vi "Run.vi"(8 "error in (no error)":errorcluster, 11 "Pub Sub Message Channel in":refnum<class "Pub Sub Message Channel.lvclass">) -> (0 "error out":errorcluster, 3 "Pub Sub Message Channel out":refnum<class "Pub Sub Message Channel.lvclass">)   [LabVIEW 2020, in "Actor Pub Sub Channels.lvlib" / "Pub Sub Message Channel.lvclass"]
uses:
  Pub Sub Message Channel.lvclass
  Close Channel Message/Close Channel Message.lvclass
  Pub Sub Message Channel.lvclass/Pub Sub Message Channel.ctl
  <vilib>/ActorFramework/Message Queue/Message Queue.lvclass/Message Queue.ctl
  <vilib>/ActorFramework/Message Dequeuer/Message Dequeuer.lvclass/Message Dequeuer.ctl
  <vilib>/ActorFramework/Message Priority Queue/Priority Dequeue.vi
  <vilib>/ActorFramework/Message Queue/Message Queue.lvclass
  <vilib>/ActorFramework/Message Dequeuer/Message Dequeuer.lvclass
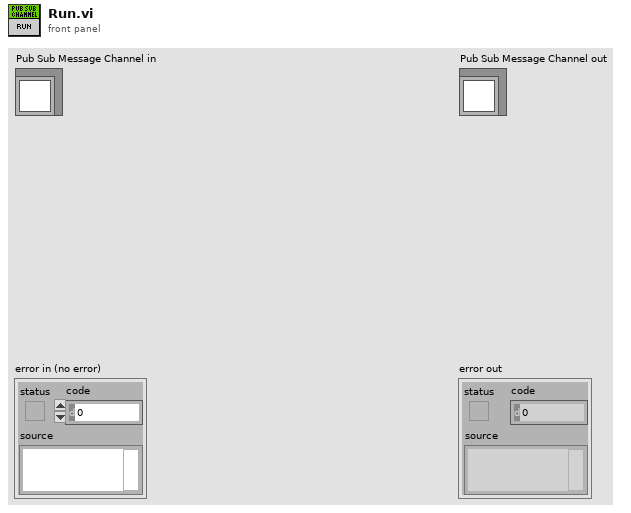
[diagram p1: front panel]
types:
  T1 = typedef "Actor Framework.lvlib/Message Dequeuer.lvclass/Dequeue Priority.ctl" = enum16{"Low", "Normal", "High", "Critical"}
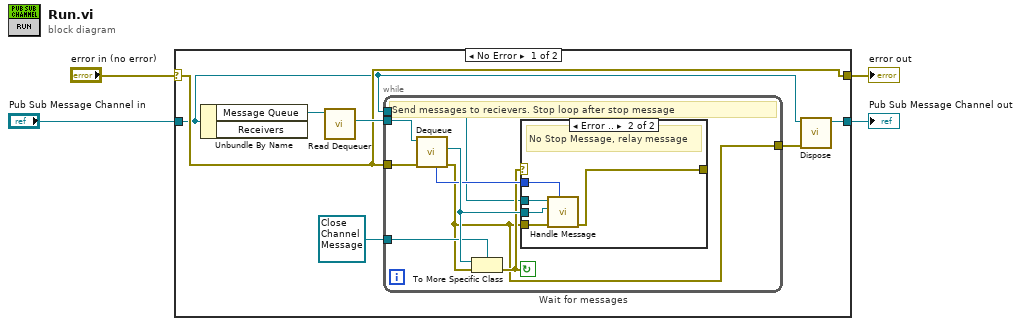
[diagram p0: block diagram]
diagram:
  n1 = case shown="No Error" "error in (no error)" {
    selector: "error in (no error)" -> [w10 w27]
    tunnel: [w10 w27] -> w3
    tunnel: [w5 w26] -> w1
    tunnel: "Pub Sub Message Channel in" -> [w6 w26]
    frame No Error {
      n2 = Unbundle By Name(w6) -> ("Message Queue"=w8:refnum<class "Message Queue.lvclass">)  [unwired: 1 out]
      n3 = call <vilib>:"Read Dequeuer.vi"("Message Queue"=w8) -> ("Message Dequeuer"=w11:refnum<class "Message Dequeuer.lvclass">)  [unwired: 10 in]
      n4 = while "Wait for messages" {
        tunnel: w11 -> [w19]
        tunnel: w10 -> [w18]
        tunnel: [w12] -> w9
        tunnel: refnum<class "Close Channel Message.lvclass"> refnum ("Actor Pub Sub Channels.lvlib:Close Channel Message.lvclass") -> [w15]
        tunnel: w6 -> [w13]
        stop <- w14 continue-if-true
        # "Send messages to recievers. Stop loop after stop message"
        n5 = call <vilib>:"Dequeue.vi"("error in (no error)"=w18, "Message Dequeuer in"=w19) -> ("error out"=w12:errorcluster, "Message"=w17:refnum<class "Message.lvclass">, "priority"=w16:T1)  [unwired: 5 in, 2 out]
        n6 = To More Specific Class(target class=w15, reference=w17, error in=w12) -> (error out=w14:errorcluster)  [unwired: 1 out]
        n7 = case shown="Error .." w14 {
          selector: w14 -> [w20 _]
          tunnel: w17 -> [_ w25]
          tunnel: w16 -> [_ w24]
          tunnel: w13 -> [_ w23]
          tunnel: [w20 w22] -> _
          tunnel: w12 -> [_ w21]
          frame No Error {
            # "stop message, dont send"
          }
          frame Error {
            # "No Stop Message, relay message"
            n8 = call-dynamic "Handle Message.vi"("priority"=w24, "error in (no error)"=w21, "Message"=w25, "Pub Sub Message Channel in"=w23) -> ("error out"=w22:errorcluster)  [unwired: 7 in]
          }
        }
      }
      n9 = call-dynamic "Dispose.vi"("error in (no error)"=w9, "Pub Sub Message Channel in"=w6) -> ("Pub Sub Message Channel in 2"=w5:refnum<class "Pub Sub Message Channel.lvclass">)  [unwired: 8 in, 1 out]
    }
    frame Error {
    }
  }
  "error out" <- w3
  "Pub Sub Message Channel out" <- w1
